vi "Shorten Cluster.vi"(3 "error in (no error)":errorcluster, 4 "Variant":variant, 5 "variable address in":string) -> (0 "error out":errorcluster, 1 "Variant":variant, 2 "variable address out":string)   [LabVIEW 2019, in "Logger.PGSQL.lvclass"]
uses:
  Logger.PGSQL.lvclass
  <vilib>/Utility/Data Type/Type Definitions/Data Type.ctl
  <vilib>/Utility/Data Type/NI_Data Type.lvlib
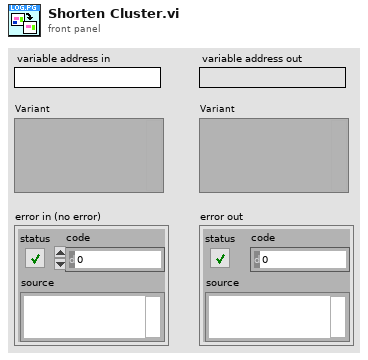
[diagram p1: front panel]
types:
  T1 = typedef "NI_Data Type.lvlib/Data Type.ctl" = enum8{"Invalid Type", "Void", "I8", "I16", "I32", "I64", "U8", "U16", "U32", "U64", "Single Float", "Double Float", "Extended Float", "Single Complex", "Double Complex", "Extended Complex", "Enum U8", "Enum U16", "Enum U32", "Enum U64", "Single Float With Unit", "Double Float With Unit", "Extended Float With Unit", "Single Complex with Unit", "Double Complex with Unit", "Extended Complex with Unit", "Boolean", "String", "Path", "Picture", "Tag", "Array", "Cluster", "Variant", "LV Variant", "Waveform", "Timestamp", "Digital Waveform", "Digital Data", "ExpressData", "Refnum", "External Data", "VI", "Poly VI", "LabVIEW Class Instance", "Fixed Point", "Set Collection", "Map Collection"}
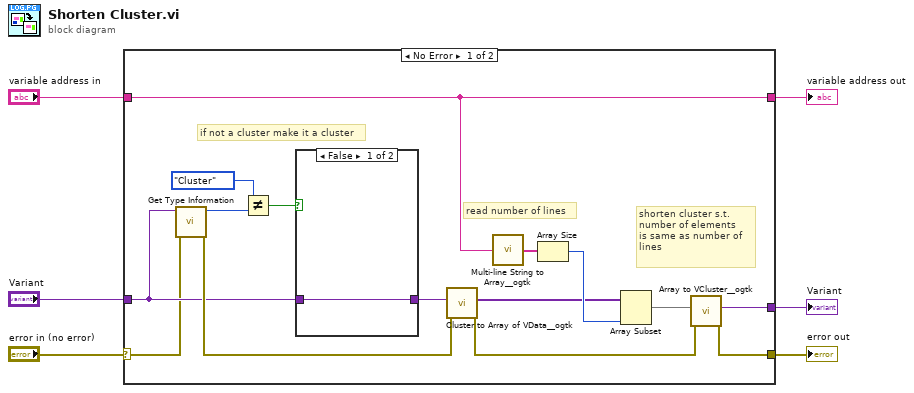
[diagram p0: block diagram]
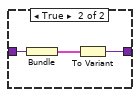
[diagram p2: hidden frame]
diagram:
  n1 = case shown="No Error" "error in (no error)" {
    selector: "error in (no error)" -> [w8 w27]
    tunnel: [w21 w27] -> w6
    tunnel: [w20 w28] -> w5
    tunnel: "variable address in" -> [w7 w26]
    tunnel: "Variant" -> [w15 w28]
    tunnel: [w7 w26] -> w1
    frame No Error {
      # "shorten cluster s.t.\nnumber of elements\nis same as number of \nlines"
      # "read number of lines"
      # "if not a cluster make it a cluster"
      n2 = call <vilib>:"Get Type Information.vi"("error in (no error)"=w8, "variant"=w15) -> ("error out"=w17:errorcluster, "type"=w19:T1)  [unwired: 5 in, 3 out]
      n3 = Not Equal?(x=Data_Type."Cluster" ("Type"), y=w19) -> (x != y?=w16:bool)
      n4 = case shown="False" w16 {
        tunnel: w15 -> [w22 w25]
        tunnel: [w22 w23] -> w14
        frame False {
        }
        frame True {
          n5 = Bundle("Variant"=w25) -> (w24:cluster{"Variant":variant})  [unwired: 1 in]
          n6 = To Variant(anything=w24) -> (Variant=w23:variant)
        }
      }
      n7 = call <userlib>:"Cluster to Array of VData__ogtk.vi"("error in (no error)"=w17, "Cluster"=w14) -> ("error out"=w9:errorcluster, "Array of VData"=w11:variant[])  [unwired: 8 in]
      n8 = call <userlib>:"Multi-line String to Array__ogtk.vi"("string"=w7) -> ("lines"=w13:string[])
      n9 = Array Size(array=w13) -> (size(s)=w12:i32)
      n10 = Array Subset(array=w11, length=w12) -> (w10:variant[])  [unwired: 1 in]
      n11 = call <userlib>:"Array to VCluster__ogtk.vi"("error in (no error)"=w9, "Array"=w10) -> ("error out"=w21:errorcluster, "VCluster"=w20:variant)  [unwired: 8 in]
    }
    frame Error {
    }
  }
  "variable address out" <- w1
  "Variant" <- w5
  "error out" <- w6
